vi "Array-Add 1D Str Column to 2D.vi"(10 "Column to Add":string[](array[string])=["7", "8", "9", "10"], 11 "Original Array":string[][](array[string])=[["1", "4"], ["2", "5"], ["3", "6"]]) -> (3 "Result Array":string[][](array[string]))   [LabVIEW 2016]
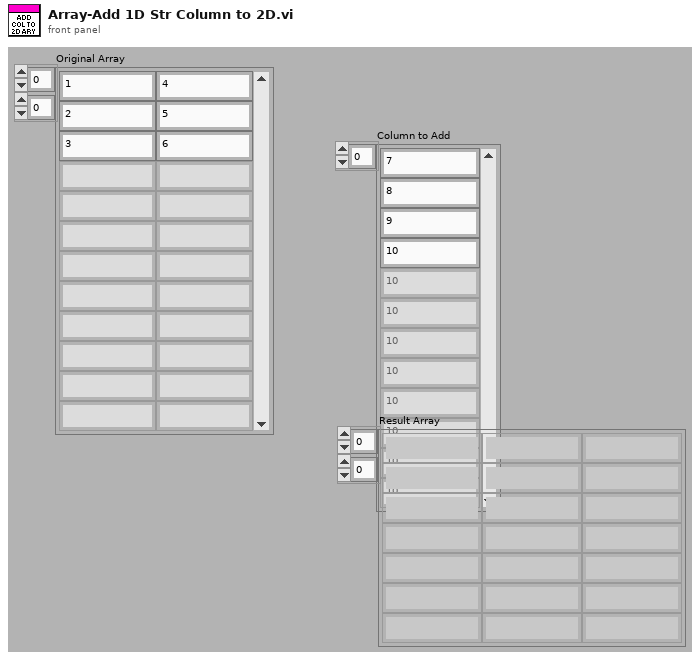
[diagram p1: front panel]
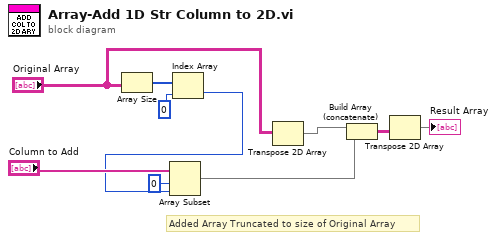
[diagram p0: block diagram]
diagram:
  # "Added Array Truncated to size of Original Array"
  n1 = Array Size(array="Original Array") -> (size(s)=w9:i32[])
  n2 = Index Array(array=w9, index=0) -> (element=w6:i32)
  n3 = Array Subset(array="Column to Add", index=0, length=w6) -> (w3:string[])
  n4 = Transpose 2D Array(2D array="Original Array") -> (transposed array=w2:string[][])
  n5 = Build Array (concatenate)(w2, w3) -> (w5:string[][])
  n6 = Transpose 2D Array(2D array=w5) -> (transposed array=→"Result Array":string[][])
